vi "originalMain.vi"(8 "error in (no error)":errorcluster) -> (0 "error out":errorcluster)   [LabVIEW 2014]
doc: "GUI for the original Actor Framework Message Maker."
uses:
  CSPP_MessageMakerMain/CS++MessageMakerMain.lvclass
  CSPP_MessageMakerMain/CS++MessageMakerMain.lvclass/CS++MessageMakerMain.ctl
  <vilib>/Utility/error.llb/Error Cluster From Error Code.vi
  <vilib>/ErrorRing/Error Ring.xnode
panel:
  out "None Found":string="No Actor classes found in this project."
  in  "Close":bool
  in  "Help":bool
  in  "Actor classes and their methods:":string[](tree)=["CS++PVProxy.lvlib:CS++PVProxy.lvclass", "CS++SVMonitor.lvlib:CS++SVMonitor.lvclass", "CS++PVMonitor.lvlib:CS++PVMonitor.lvclass", "CS++DeviceActor.lvlib:CS++DeviceActor.lvclass"]
  in  "Build Selected":bool
  in  "Projects":u16(ring) caption="Project to display:"
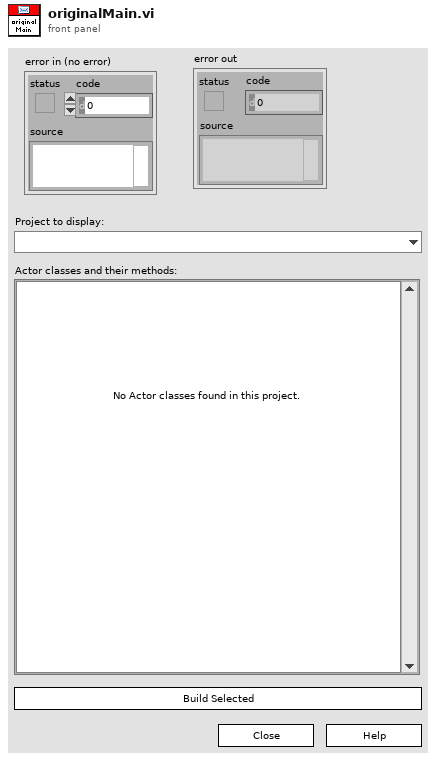
[diagram p1: front panel]
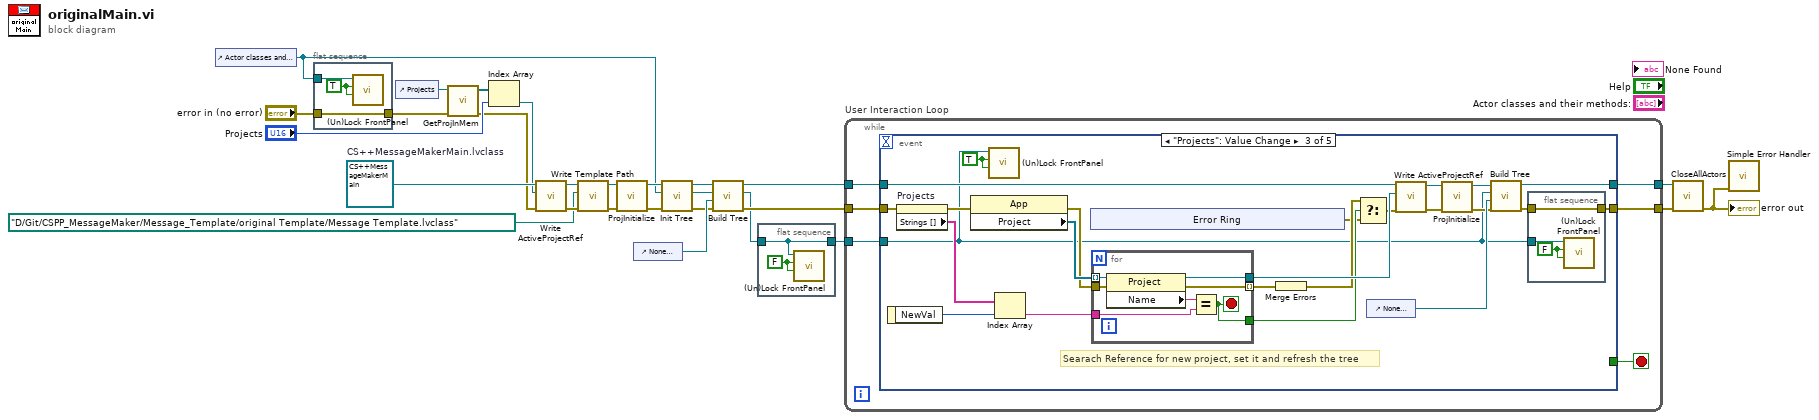
[diagram p0: block diagram]
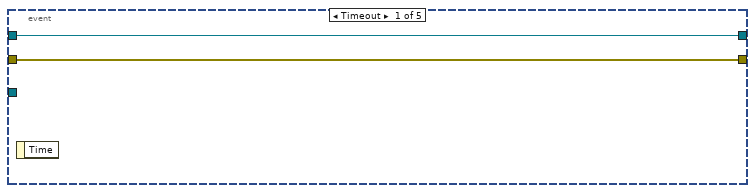
[diagram p2: hidden frame]
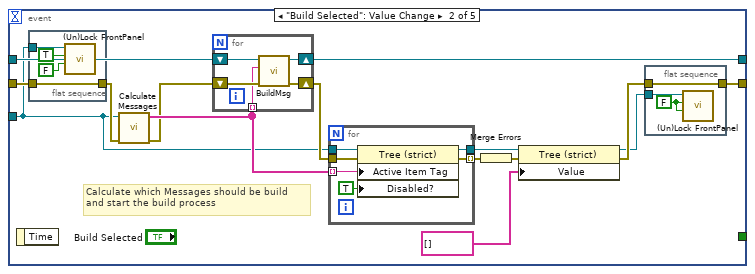
[diagram p3: hidden frame]
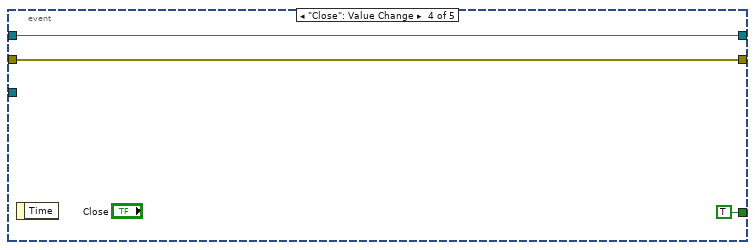
[diagram p4: hidden frame]
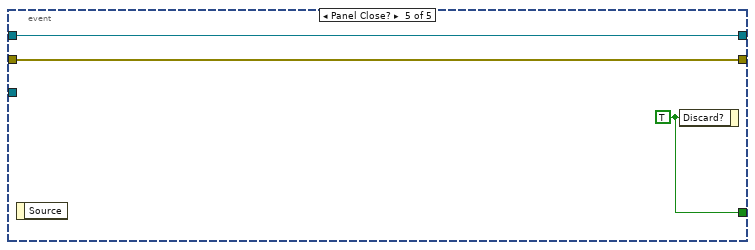
[diagram p5: hidden frame]
diagram:
  w27 = refnum<class "CS++MessageMakerMain.lvclass"> refnum  # CS++MessageMakerMain.lvclass
  n1 = control-ref of="Actor classes and their methods:"() -> (w3:refnum<vi>)
  n2 = flat-sequence {
    tunnel: w3 -> [w30]
    tunnel: "error in (no error)" -> [w29]
    tunnel: [w29] -> w1
    frame #0 {
      w28 = TRUE
      n3 = call "(Un)Lock FrontPanel.vi"("SetDeferPanel?"=w28, "Lock?"=w28, "Tree Reference"=w30) -> ()  [unwired: 9 in]
    }
  }
  n4 = control-ref of="Projects"() -> (w26:refnum<vi>)
  n5 = call "GetProjInMem.vi"("error in (no error)"=w1, "Ring refnum"=w26) -> ("error out"=w22:errorcluster, "Project:Projects[]"=w25:refnum<vi>[])  [unwired: 8 in]
  n6 = Index Array(array=w25, index="Projects") -> (element=w23:refnum<vi>)
  n7 = call "Write ActiveProjectRef.vi"("error in (no error)"=w22, "ActiveProjectRef"=w23, "CS++MessageMakerMain in"=w27) -> ("error out"=w16:errorcluster, "CS++MessageMakerMain out"=w17:refnum<class "CS++MessageMakerMain.lvclass">)  [unwired: 7 in]
  n8 = call "Write Template Path.vi"("error in (no error)"=w16, "Template Path"=path "D:/Git/CSPP_MessageMaker/Message_Template/original Template/Message Template.lvclass", "CS++MessageMakerMain in"=w17) -> ("error out"=w15:errorcluster, "CS++MessageMakerMain out"=w18:refnum<class "CS++MessageMakerMain.lvclass">)  [unwired: 7 in]
  n9 = call-dynamic "ProjInitialize.vi"("error in (no error)"=w15, "CS++MessageMakerMain in"=w18) -> ("error out"=w5:errorcluster, "CS++MessageMakerMain out"=w7:refnum<class "CS++MessageMakerMain.lvclass">)  [unwired: 8 in]
  n10 = control-ref of="None Found"() -> (w12:refnum<vi>)
  n11 = call "Init Tree.vi"("error in (no error)"=w5, "Tree Reference In"=w3, "CS++MessageMakerMain in"=w7) -> ("error out"=w8:errorcluster, "Tree Reference Out"=w4:refnum<vi>, "CS++MessageMakerMain out"=w6:refnum<class "CS++MessageMakerMain.lvclass">)  [unwired: 6 in]
  n12 = call "Build Tree.vi"("error in (no error)"=w8, "No Project Text Reference"=w12, "Tree Reference In"=w4, "CS++MessageMakerMain in"=w6) -> ("error out"=w11:errorcluster, "Tree Reference Out"=w9:refnum<vi>, "CS++MessageMakerMain out"=w13:refnum<class "CS++MessageMakerMain.lvclass">)  [unwired: 5 in]
  n13 = flat-sequence {
    tunnel: [w31] -> w10
    tunnel: w9 -> [w31]
    frame #0 {
      w32 = FALSE
      n14 = call "(Un)Lock FrontPanel.vi"("SetDeferPanel?"=w32, "Lock?"=w32, "Tree Reference"=w31) -> ()  [unwired: 9 in]
    }
  }
  n15 = while "User Interaction Loop" {
    tunnel: w11 -> [w38]
    tunnel: [w37] -> w21
    tunnel: w13 -> [w33]
    tunnel: [w35] -> w19
    tunnel: w10 -> [w34]
    stop <- w36 stop-if-true
    n16 = event shown="[2] \"Projects\": Value Change" {
      selector: _ -> [_ _ _ _ _]
      dyn-events: _ -> [_ _ _ _ _]
      timeout: _ -> [_ _ _ _ _]
      tunnel: w38 -> [w40 w44 w94 w114 w115]
      tunnel: [w40 w55 w77 w114 w115] -> w37
      tunnel: [_ _ _ TRUE w117] -> w36
      tunnel: w33 -> [w39 w45 w89 w112 w116]
      tunnel: [w39 w50 w97 w112 w116] -> w35
      tunnel: w34 -> [_ w41 w74 _ _]
      event Timeout {
        n17 = event-data() -> ()  [unwired: 1 in, 1 out]
      }
      event "Build Selected": Value Change {
        # "Calculate which Messages should be build\nand start the build process"
        n18 = event-data() -> ()  [unwired: 1 in, 1 out]
        n19 = flat-sequence {
          tunnel: w44 -> [w57]
          tunnel: [w57] -> w43
          tunnel: w41 -> [w56]
          frame #0 {
            n20 = call "(Un)Lock FrontPanel.vi"("SetDeferPanel?"=FALSE, "Lock?"=TRUE, "Tree Reference"=w56) -> ()  [unwired: 9 in]
          }
        }
        n21 = call "Calculate Messages.vi"("error in (no error)"=w43, "Tree Reference"=w41) -> ("error out"=w46:errorcluster, "Array of Messages to be build"=w53:string[])  [unwired: 8 in]
        n22 = for {
          shift-right: [w67] -> w54
          shift-left: w46 -> [w69]
          shift-right: [w70] -> w50
          shift-left: w45 -> [w68]
          tunnel: w53 -> [w66] mode=indexing
          n23 = call "BuildMsg.vi"("error in (no error)"=w69, "Msg to be build"=w66, "CS++MessageMakerMain in"=w68) -> ("error out"=w67:errorcluster, "CS++MessageMakerMain out"=w70:refnum<class "CS++MessageMakerMain.lvclass">)  [unwired: 7 in]
        }
        n24 = for {
          tunnel: w41 -> [w65]
          tunnel: w54 -> [w64]
          tunnel: w53 -> [w63] mode=indexing
          tunnel: [w61] -> w49 mode=indexing
          tunnel: [w60] -> w52
          n25 = property class="Tree (strict)"(reference=w65, error in=w64, "Active Item Tag"=w63, "Disabled?"=TRUE ("Active Item:Disabled?")) -> (reference out=w60:refnum<vi>, error out=w61:errorcluster)
        }
        n26 = Merge Errors(w49) -> (w48:errorcluster)
        n27 = property class="Tree (strict)"(reference=w52, error in=w48, "Value"=string[] []) -> (reference out=w42:refnum<vi>, error out=w51:errorcluster)
        n28 = flat-sequence {
          tunnel: [w73] -> w55
          tunnel: w51 -> [w73]
          tunnel: w42 -> [w71]
          frame #0 {
            w72 = FALSE
            n29 = call "(Un)Lock FrontPanel.vi"("SetDeferPanel?"=w72, "Lock?"=w72, "Tree Reference"=w71) -> ()  [unwired: 9 in]
          }
        }
      }
      event "Projects": Value Change {
        w75 = TRUE
        # "Searach Reference for new project, set it and refresh the tree"
        n30 = event-data() -> ("NewVal"=w92:u16)  [unwired: 1 in]
        n31 = property on="Projects" class="Ring (strict)"(error in=w94) -> (error out=w78:errorcluster, "Strings []"=w93:string[])  [unwired: 1 in, 1 out]
        n32 = property class="App"(error in=w78) -> (error out=w95:errorcluster, "Project"=w96:refnum<vi>[])  [unwired: 1 in, 1 out]
        n33 = call "(Un)Lock FrontPanel.vi"("SetDeferPanel?"=w75, "Lock?"=w75, "Tree Reference"=w74) -> ()  [unwired: 9 in]
        n34 = Index Array(array=w93, index=w92) -> (element=w91:string)
        n35 = xnode "Error Ring"() -> ("error out"=w85:errorcluster)
        n36 = for {
          tunnel: w96 -> [w111] mode=indexing
          tunnel: w95 -> [w110]
          tunnel: [w109] -> w87 mode=indexing
          tunnel: [w107] -> w90
          tunnel: w91 -> [w106]
          tunnel: [w105] -> w88
          stop <- w105 stop-if-true
          n37 = property class="Project"(reference=w111, error in=w110) -> (reference out=w107:refnum<vi>, error out=w109:errorcluster, "Name"=w108:string)
          n38 = Equal?(x=w108, y=w106) -> (x = y?=w105:bool)
        }
        n39 = Merge Errors(w87) -> (w86:errorcluster)
        n40 = Select(t=w86, s=w88, f=w85) -> (s? t:f=w84:errorcluster)
        n41 = control-ref of="None Found"() -> (w83:refnum<vi>)
        n42 = call "Write ActiveProjectRef.vi"("error in (no error)"=w84, "ActiveProjectRef"=w90, "CS++MessageMakerMain in"=w89) -> ("error out"=w80:errorcluster, "CS++MessageMakerMain out"=w82:refnum<class "CS++MessageMakerMain.lvclass">)  [unwired: 7 in]
        n43 = call-dynamic "ProjInitialize.vi"("error in (no error)"=w80, "CS++MessageMakerMain in"=w82) -> ("error out"=w79:errorcluster, "CS++MessageMakerMain out"=w81:refnum<class "CS++MessageMakerMain.lvclass">)  [unwired: 8 in]
        n44 = call "Build Tree.vi"("error in (no error)"=w79, "No Project Text Reference"=w83, "Tree Reference In"=w74, "CS++MessageMakerMain in"=w81) -> ("error out"=w76:errorcluster, "CS++MessageMakerMain out"=w97:refnum<class "CS++MessageMakerMain.lvclass">)  [unwired: 5 in, 1 out]
        n45 = flat-sequence {
          tunnel: [w100] -> w77
          tunnel: w76 -> [w100]
          tunnel: w74 -> [w98]
          frame #0 {
            w99 = FALSE
            n46 = call "(Un)Lock FrontPanel.vi"("SetDeferPanel?"=w99, "Lock?"=w99, "Tree Reference"=w98) -> ()  [unwired: 9 in]
          }
        }
      }
      event "Close": Value Change {
        n47 = event-data() -> ()  [unwired: 1 in, 1 out]
      }
      event Panel Close? {
        w117 = TRUE ("Discard?")
        n48 = event-data() -> ()  [unwired: 1 in, 1 out]
        n49 = event-data("Discard?"=w117) -> ()  [unwired: 1 in, 1 out]
      }
    }
  }
  n50 = call-dynamic "CloseAllActors.vi"("error in (no error)"=w21, "CS++MessageMakerMain in"=w19) -> ("error out"=w20:errorcluster)  [unwired: 8 in, 1 out]
  "error out" <- w20
  n51 = call <vilib>:"Simple Error Handler.vi"("error in (no error)"=w20) -> ()  [unwired: 4 in, 5 out]
